vi "Create Message Channel.vi"(8 "error in (no error)":errorcluster) -> (0 "error out":errorcluster, 3 "Message Channel":refnum<user-event>)   [LabVIEW 2020, in "RTAF.lvlib" / "Actor.lvclass"]
uses:
  Actor.lvclass
  Message.ctl
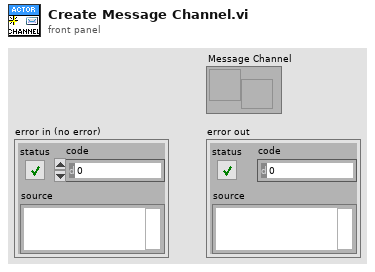
[diagram p1: front panel]
types:
  T1 = typedef "RTAF.lvlib/Actor.lvclass/Message.ctl" = cluster{"Name":string, "Payload":variant, "Response Channel":refnum<notifier>}
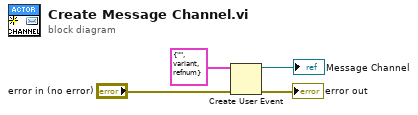
[diagram p0: block diagram]
diagram:
  n1 = Create User Event(user event datatype=T1 {"Name"="", "Payload"=variant, "Response Channel"=refnum} ("Message"), error in="error in (no error)") -> (user event=→"Message Channel":refnum<user-event>, error out=→"error out":errorcluster)
